vi "RobotSimulator.vi"() -> ()   [LabVIEW 2018]
uses:
  Robot-Project/Drive/Implementation/Drive Setpoints.ctl
  Robot-Project/Drive/Implementation/Drive Operations.ctl
  Controls/PurePursuit/RobotNeededPathData.ctl
  Robot-Project/Drive/DriveState.ctl
  <extravilib>/ChannelInstances/Lossy Stream-c(dbl,dbl,dbl,c(dbl,dbl))/Write With Abort.vi
  <extravilib>/ChannelInstances/Lossy Stream-c(dbl,dbl,dbl,c(dbl,dbl))/Read With Abort.vi
  <extravilib>/ChannelInstances/Lossy Stream-c(dbl,dbl,dbl,c(dbl,dbl))/Endpoint.vi
  <extravilib>/ChannelInstances/Lossy Stream-c(dbl,dbl,dbl,c(dbl,dbl))/EndpointRead.vi
  Robot-Project/Drive/Implementation/Drive Published Globals.vi
  <extravilib>/ChannelInstances/Lossy Stream-c(dbl,dbl,dbl,c(dbl,dbl))/Instantiate.vi
  <extravilib>/ChannelInstances/Lossy Stream-c(dbl,dbl,dbl,c(dbl,dbl))/)Channel.vi
  <resource>/ChannelSupport/_ChannelSupport/WaitIfNeeded.vi
  <vilib>/addons/control/pid/pid.llb/PID (DBL).vi
  Robot-Project/Configuration/Constants.vi
  <vilib>/addons/control/pid/NI_PID_pid.lvlib
  <extravilib>/ChannelInstances/Lossy Stream-c(dbl,dbl,dbl,c(dbl,dbl)).lvlib
panel:
  in  "Path":cluster{dbl, dbl}[](array[cluster])
  in  "Angle Addition":dbl(slide) scale=-180.0..180.0
  in  "Target":cluster{dbl, dbl}={200.0, 200.0}
  out "Current\nCmd":string="Started at  14:51:47.884\nDefault: Reserve,  L 0.0, R 0.0, D 0.000000"
  in  "Go":bool
  out "Loop Iterations":i32
  in  "Gains 2":T1={"Gains"={"FFV"=0.0055, "FFA"=0.0025, "Vel PID"={"P"=0.05, "I"=0.0, "D"=0.0}}, "Pos PID"={"P"=0.05, "I"=0.0, "D"=0.0}, "MinVoltage"=0.0, "Effective Trackwidth"=29.0, "Effective Trackwidth CCW"=29.0} {"Pos PID"."D" format="%.3f"; "Pos PID"."I" format="%.3f"; "Pos PID"."P" format="%.3f"; "Gains"."Vel PID"."D" format="%.3f"; "Gains"."Vel PID"."I" format="%.3f"; "Gains"."Vel PID"."P" format="%.3f"}
  out "Graph":cluster{cluster{"x":dbl, "y":dbl}[]}[](graph)=[{[]}, {[{"x"=19.5, "y"=127.60329985652797}, {"x"=31.499289530461766, "y"=127.73387843115106}]}, {[{"x"=0.0, "y"=0.0}]}, {[{"x"=19.5, "y"=127.60329985652797}, {"x"=19.5, "y"=127.60329985652797}, {"x"=19.5, "y"=127.60329985652797}, {"x"=19.5, "y"=127.60329985652797}, {"x"=19.5, "y"=127.60329985652797}, {"x"=19.5, "y"=127.60329985652797}, {"x"=19.5, "y"=127.60329985652797}, {"x"=19.5, "y"=127.60329985652797}, {"x"=19.5, "y"=127.60329985652797}, {"x"=19.5, "y"=127.60329985652797}, {"x"=19.5, "y"=127.60329985652797}, {"x"=19.5, "y"=127.60329985652797}, {"x"=19.5, "y"=127.60329985652797}, {"x"=19.5, "y"=127.60329985652797}, {"x"=19.5, "y"=127.60329985652797}, {"x"=19.5, "y"=127.60329985652797}, {"x"=19.5, "y"=127.60329985652797}, {"x"=19.5, "y"=127.60329985652797}, {"x"=19.5, "y"=127.60329985652797}, {"x"=19.5, "y"=127.60329985652797}, {"x"=19.5, "y"=127.60329985652797}, {"x"=19.5, "y"=127.60329985652797}, {"x"=19.5, "y"=127.60329985652797}, {"x"=19.5, "y"=127.60329985652797}, {"x"=19.5, "y"=127.60329985652797}, {"x"=19.5, "y"=127.60329985652797}, {"x"=19.5, "y"=127.60329985652797}, {"x"=19.5, "y"=127.60329985652797}, {"x"=19.5, "y"=127.60329985652797}, {"x"=19.5, "y"=127.60329985652797}, {"x"=19.5, "y"=127.60329985652797}]}, {[{"x"=inf, "y"=nan}, {"x"=inf, "y"=nan}, {"x"=inf, "y"=nan}, {"x"=inf, "y"=nan}, {"x"=inf, "y"=nan}, {"x"=inf, "y"=nan}, {"x"=inf, "y"=nan}, {"x"=inf, "y"=nan}, {"x"=nan, "y"=nan}, {"x"=nan, "y"=nan}, {"x"=nan, "y"=nan}, {"x"=nan, "y"=nan}, {"x"=nan, "y"=nan}, {"x"=nan, "y"=nan}, {"x"=nan, "y"=nan}, {"x"=nan, "y"=nan}, {"x"=nan, "y"=-inf}, {"x"=nan, "y"=-inf}, {"x"=nan, "y"=-inf}, {"x"=nan, "y"=-inf}, {"x"=nan, "y"=-inf}, {"x"=nan, "y"=-inf}, {"x"=nan, "y"=-inf}, {"x"=inf, "y"=-inf}, {"x"=inf, "y"=-inf}, {"x"=inf, "y"=-inf}, {"x"=inf, "y"=-inf}, {"x"=inf, "y"=-inf}, {"x"=inf, "y"=-inf}, {"x"=inf, "y"=-inf}, {"x"=inf, "y"=-inf}]}]
  out "Right Output":dbl
  out "Left Output":dbl
  in  "Config":T2={"Gear Reduction"=8.7, "Wheel Radius (m)"=0.076, "# Motors"=3, "coeff of friction"=0.1, "Mass (kg)"=55.0, "Motor"={"Ke (V)"=0.0183, "R (ohms)"=0.14, "KT (Nm/A)"=0.0183, "Tf (Nm)"=0.015}}
  in  "Position":dbl=3.0
  in  "Gains":T3={"FFV"=0.0059, "FFA"=0.0019, "Vel PID"={"P"=0.01, "I"=0.0, "D"=0.0}}
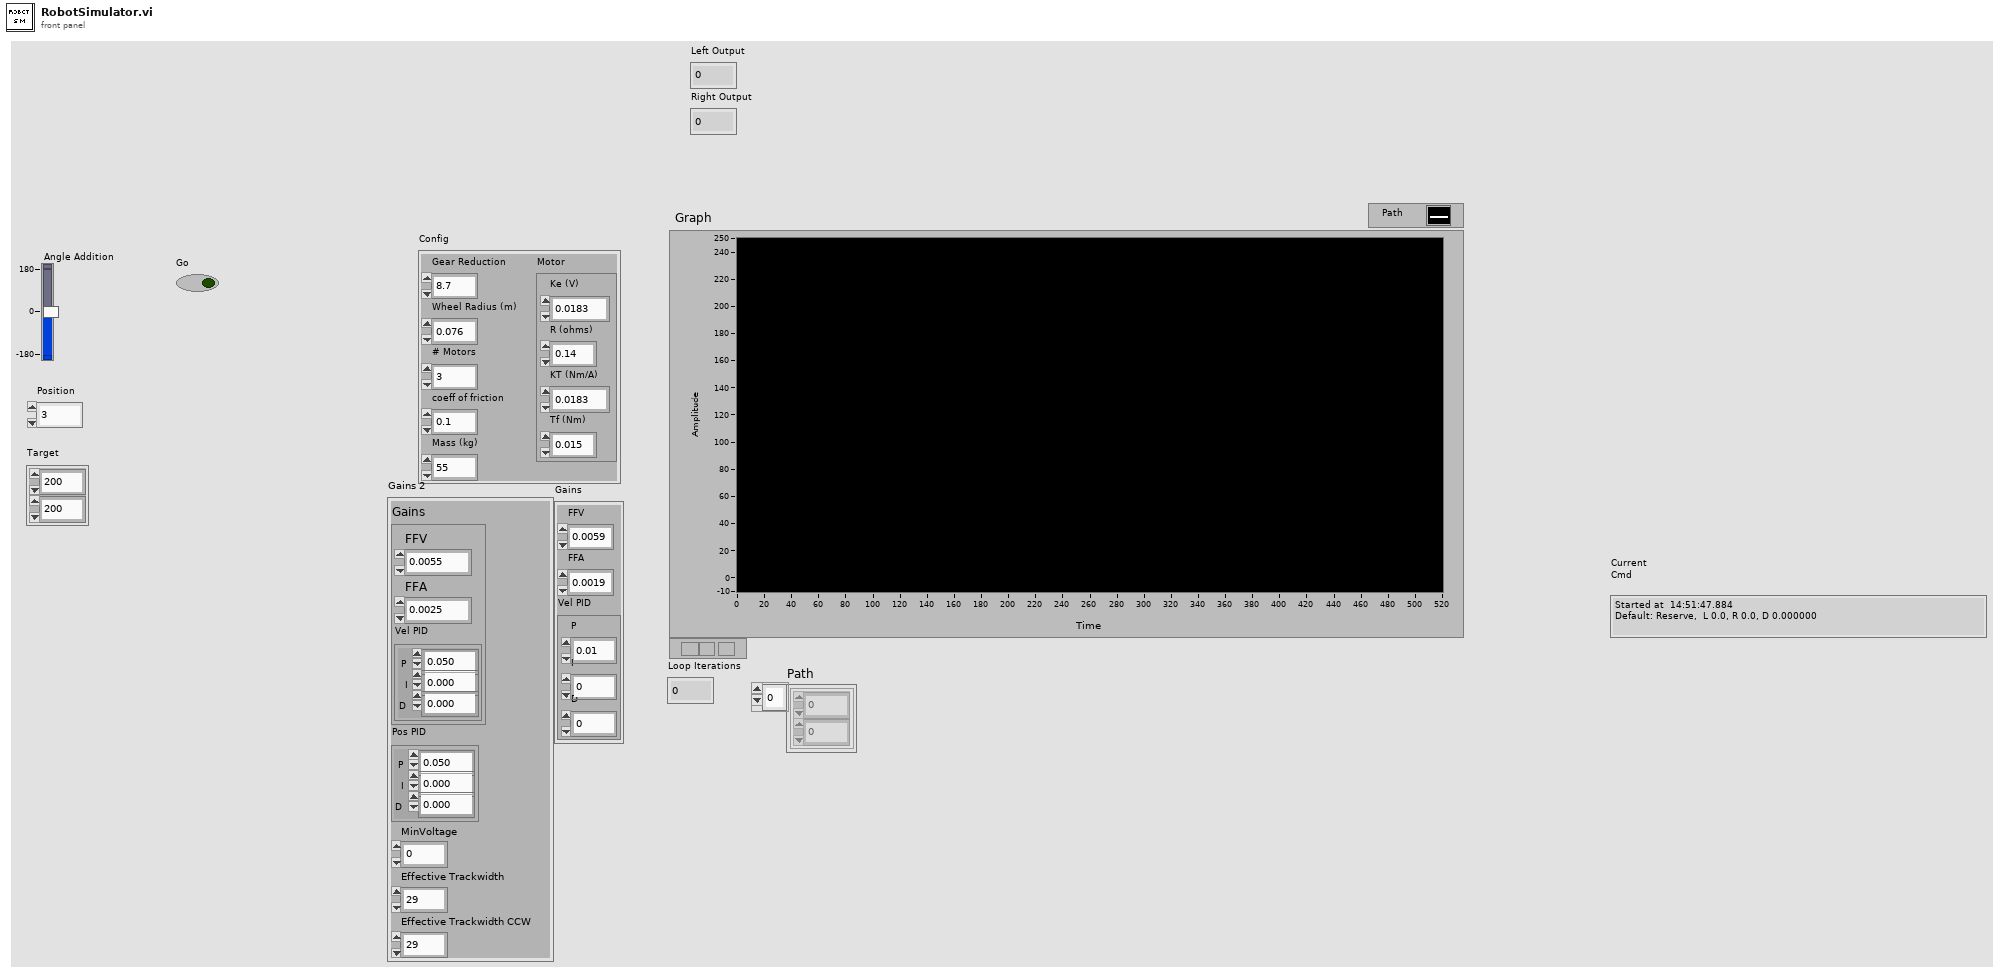
[diagram p1: front panel]
types:
  T1 = cluster{"Gains":cluster{"FFV":dbl, "FFA":dbl, "Vel PID":cluster{"P":dbl, "I":dbl, "D":dbl}}, "Pos PID":cluster{"P":dbl, "I":dbl, "D":dbl}, "MinVoltage":dbl, "Effective Trackwidth":dbl, "Effective Trackwidth CCW":dbl}
  T2 = cluster{"Gear Reduction":dbl, "Wheel Radius (m)":dbl, "# Motors":u32, "coeff of friction":dbl, "Mass (kg)":dbl, "Motor":cluster{"Ke (V)":dbl, "R (ohms)":dbl, "KT (Nm/A)":dbl, "Tf (Nm)":dbl}}
  T3 = cluster{"FFV":dbl, "FFA":dbl, "Vel PID":cluster{"P":dbl, "I":dbl, "D":dbl}}
  T4 = typedef "Drive Setpoints.ctl" = cluster{"Operation":T5, "Left Speed":dbl, "Right Speed":dbl, "Duration":dbl, "Speed":dbl, "Start Angle":dbl, "Target Angle":dbl, "Distance (inch)":dbl, "Start Point (inch)":dbl, "RobotNeededPathData":T6, "Start Point 2":dbl}
  T5 = typedef "Drive Operations.ctl" = enum16{"Reserve", "Read Current", "Immediate", "Drive for Time", "Drive for Distance", "Turn to Angle", "Drive Path"}
  T6 = typedef "RobotNeededPathData.ctl" = cluster{"Path":cluster{dbl, dbl}[], "MaxVel":dbl, "MaxAccel":dbl, "Backwards?":bool, "PointSpacing":dbl, "LookaheadDist":dbl, "Speed/Curve":dbl, "SlowDistanceAtEnd":dbl, "SlowSpeed":dbl, "MaxDeAccel":dbl}
  T7 = typedef "Command Status Info.ctl" = cluster{"Name":string, "Status":T8, "notifier out":T9}
  T8 = typedef "Completion Status.ctl" = enum16{"Successful", "Aborted", "Incomplete"}
  T9 = typedef "Completion Notifier.ctl" = refnum<notifier>
  T10 = cluster{"SubSystem Data":T4, cluster{"Start Time (ms)":u32, "Iterations":i32}, cluster{"Command Info":T7, "Description":string, "Default Command":T4, "queue out":refnum<queue>, "Subsystem Name":string}}
  T11 = typedef "DriveState.ctl" = enum16{"None", "Initial Turn", "Follow Path"}
  T12 = cluster{"LeftVel":dbl, "RightVel":dbl, "Yaw":dbl, "Pos":cluster{"X":dbl, "Y":dbl}}
  T13 = typedef "Lossy Stream-c(dbl,dbl,dbl,c(dbl,dbl)).lvlib/)Channel.ctl" = refnum<queue>
  T14 = cluster{"proportional gain (Kc)":dbl, "integral time (Ti, min)":dbl, "derivative time (Td, min)":dbl}
  T15 = cluster{"Angle":dbl, "Angular vel":dbl, "Left Distance":dbl, "Left vel":dbl, "Right Distance":dbl, "Right vel":dbl}
  T16 = cluster{"LeftDistance":dbl, "RightDistance":dbl, "LeftVelocity":dbl, "RightVelocity":dbl, "Angle":dbl, "Location":cluster{dbl, dbl}}
  T17 = cluster{"dx/dt":dbl, "dx/dt":dbl, "Yaw":dbl, cluster{dbl, dbl}}
  T18 = cluster{"SubSystem Data":T4, cluster{"Start Time (ms)":u32, "Iterations":i32}, "Default Command Arguments":cluster{"Command Info":T7, "Description":string, "Default Command":T4, "queue out":refnum<queue>, "Subsystem Name":string}}
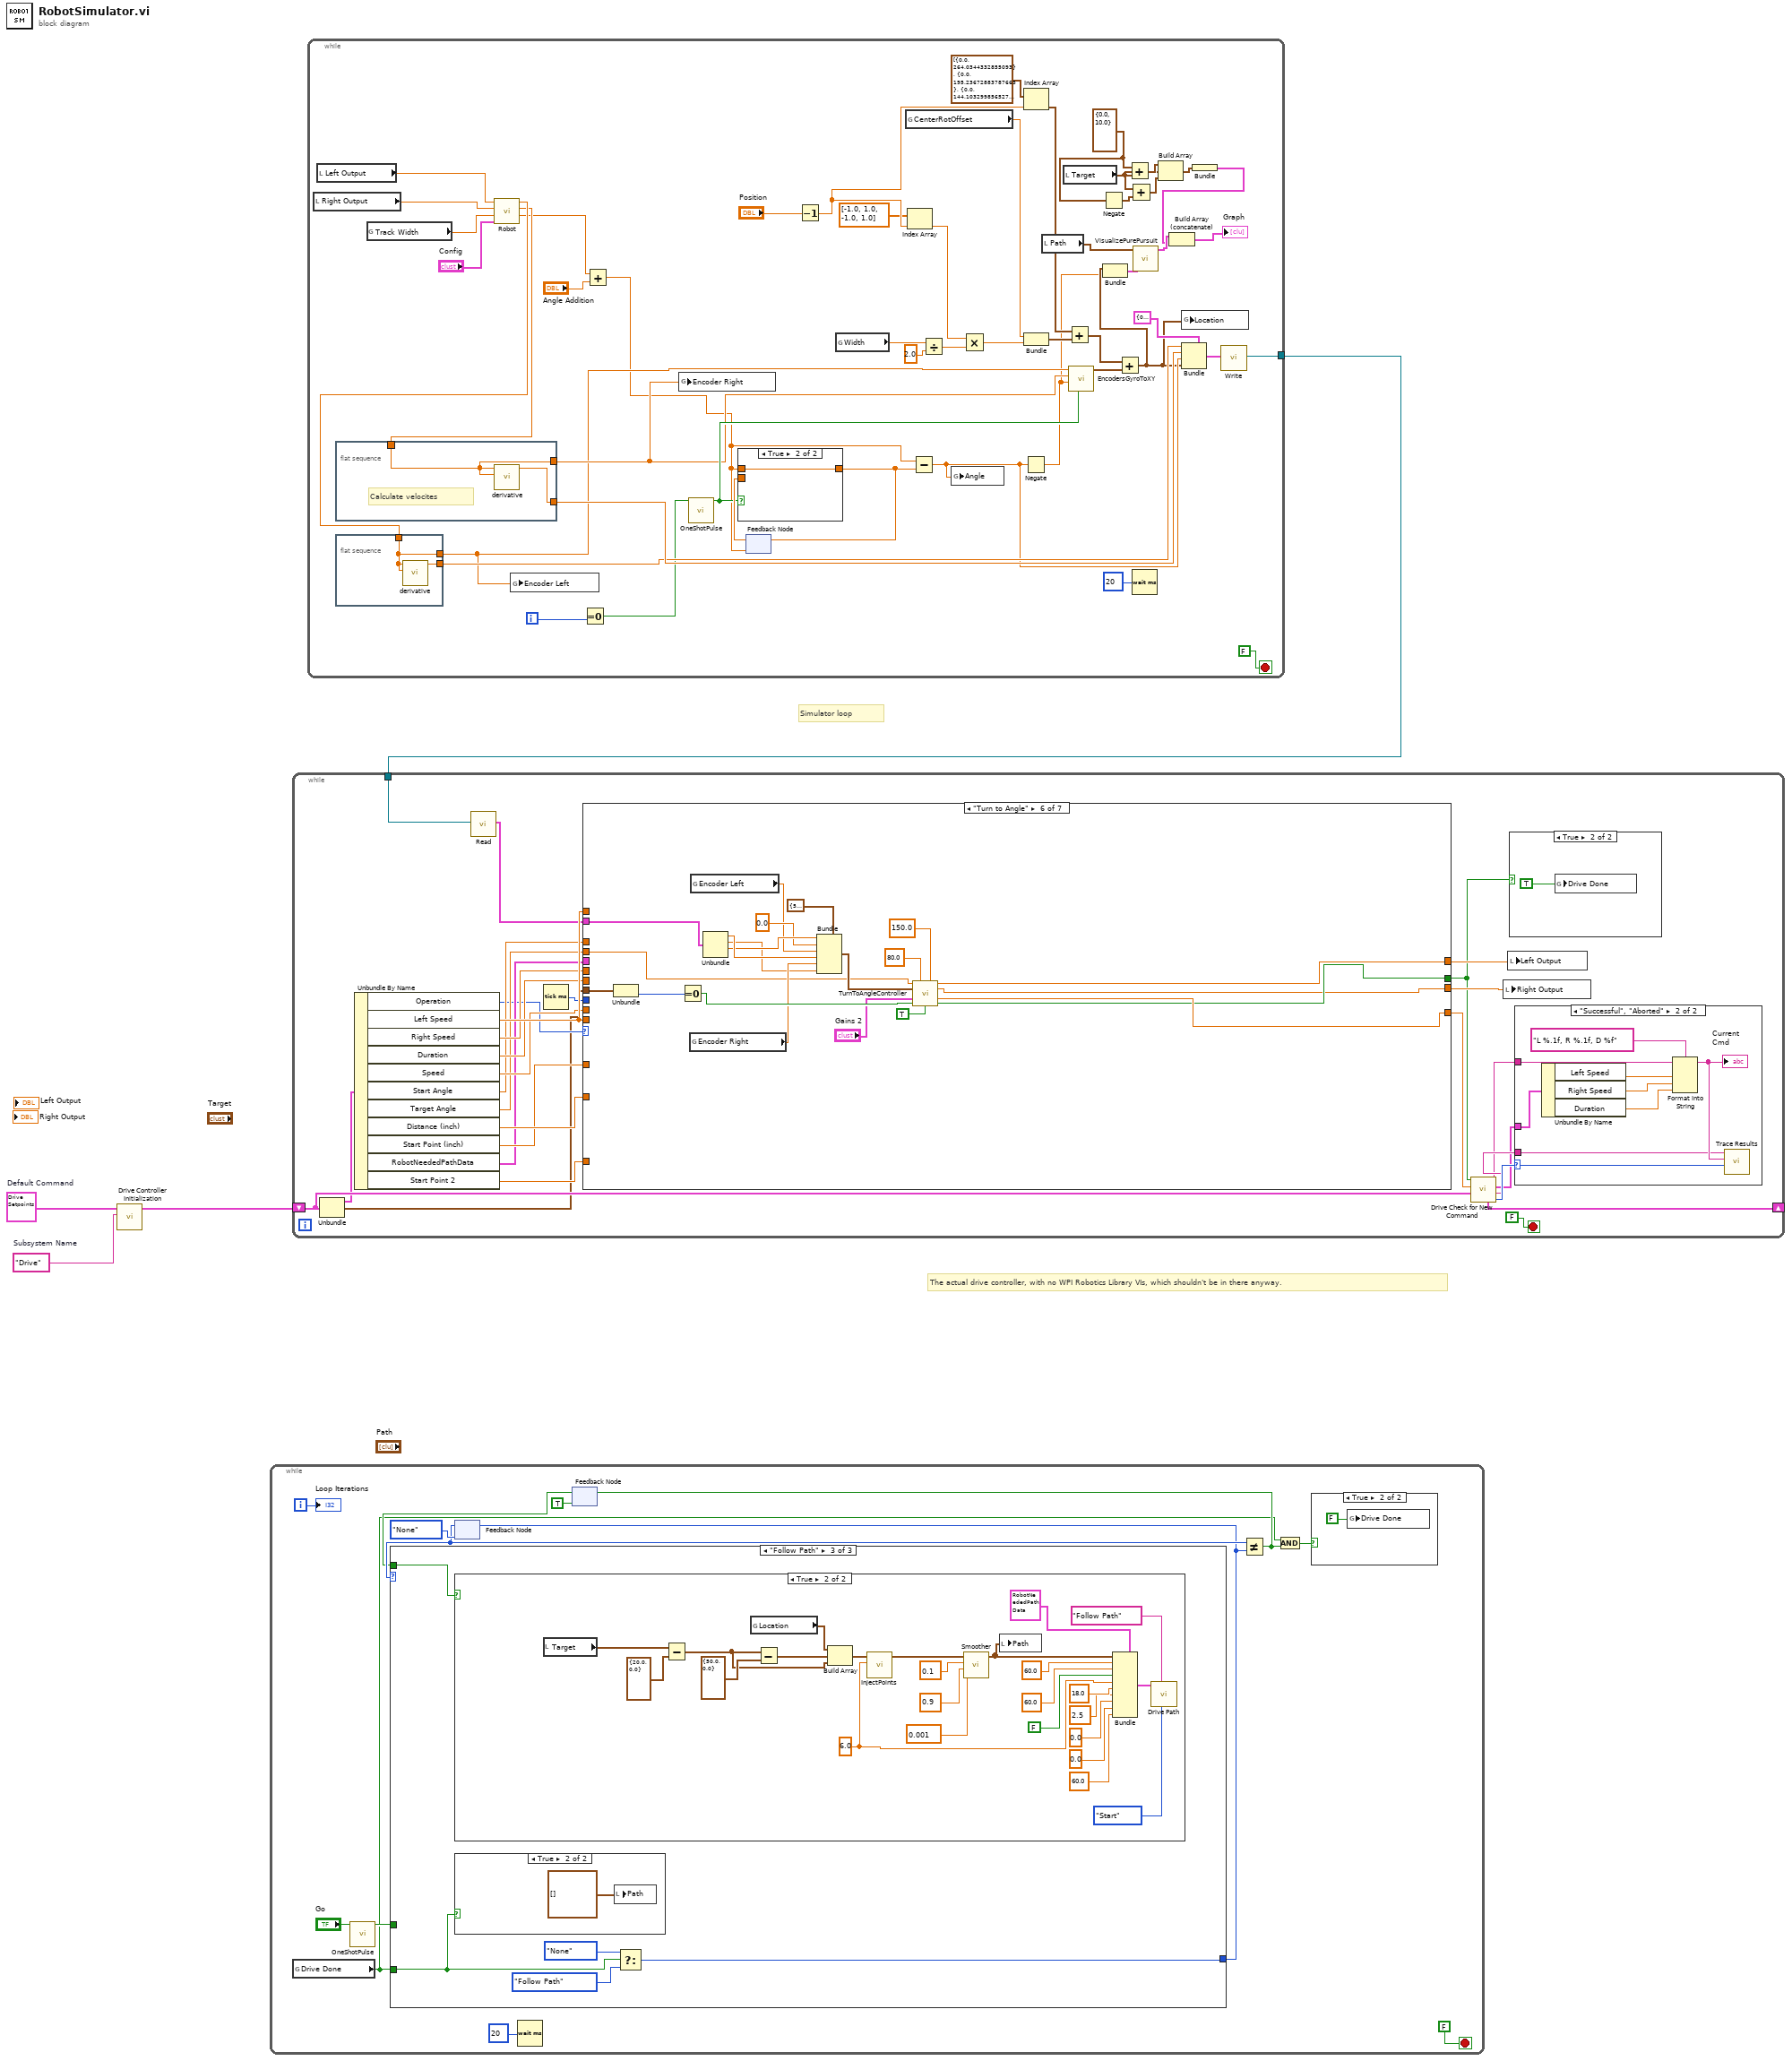
[diagram p0: block diagram]
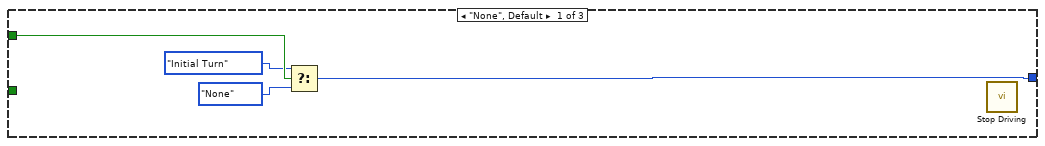
[diagram p3: hidden frame]
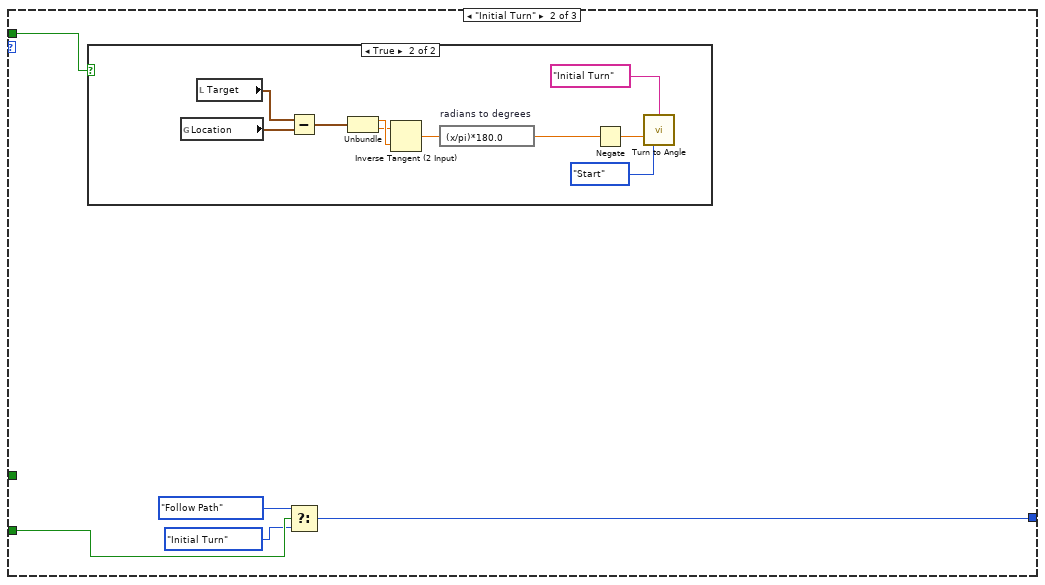
[diagram p4: hidden frame]
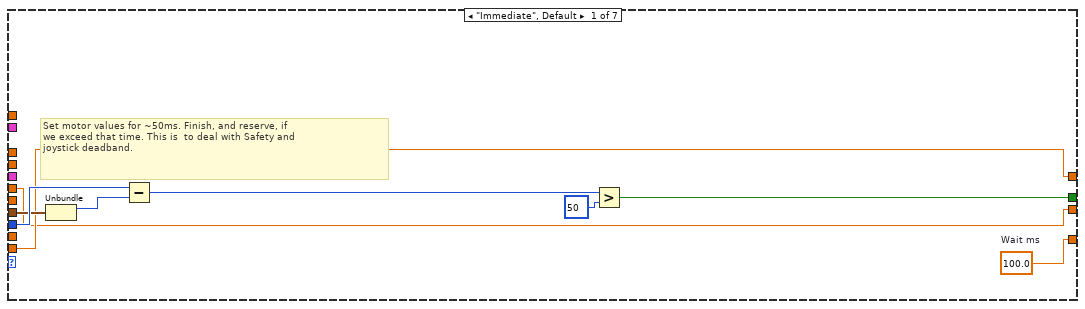
[diagram p11: hidden frame]
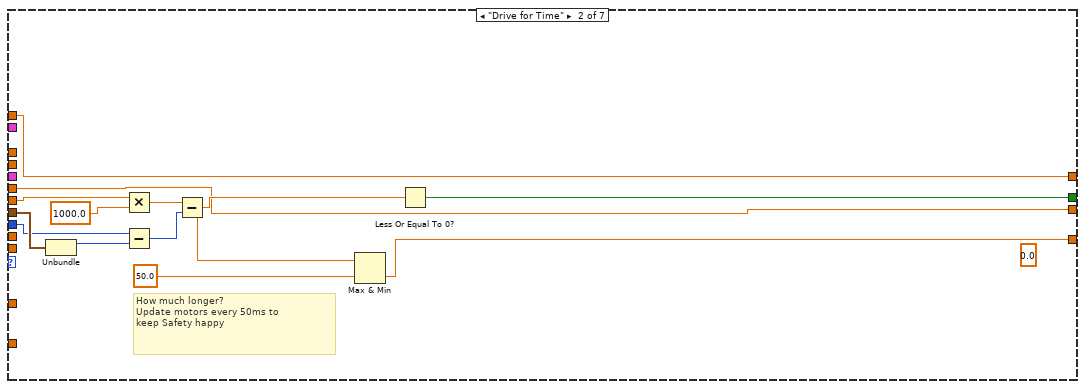
[diagram p12: hidden frame]
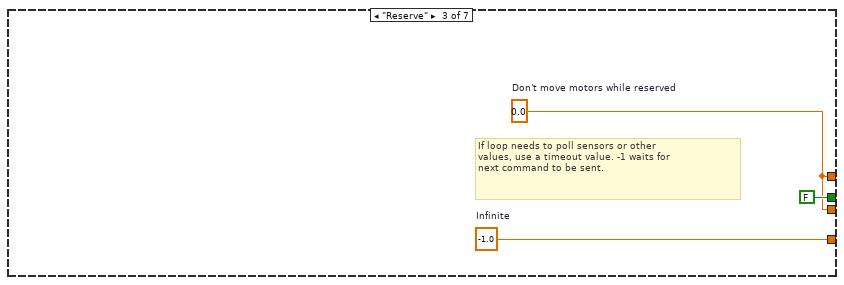
[diagram p13: hidden frame]
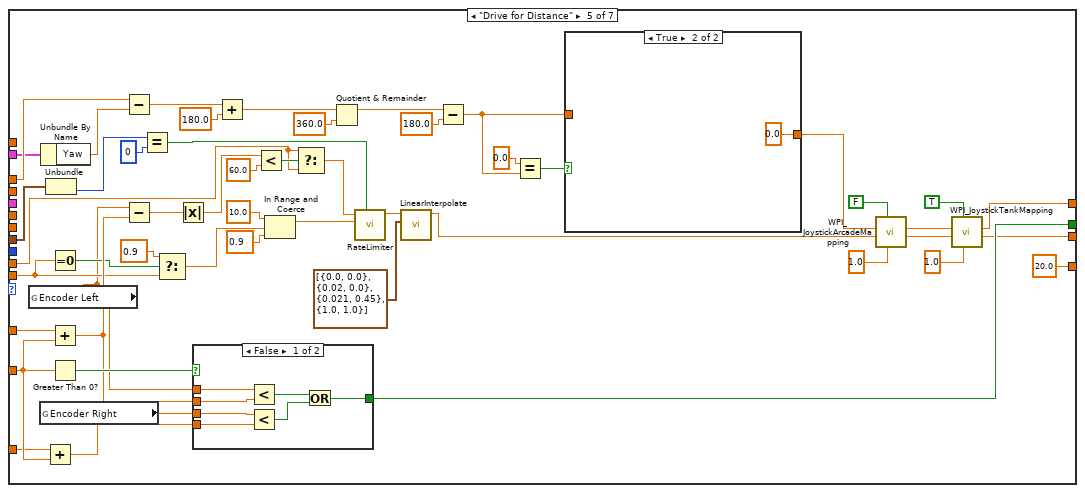
[diagram p15: hidden frame]
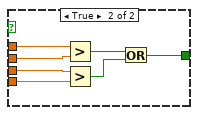
[diagram p16: hidden frame]
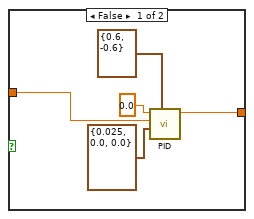
[diagram p17: hidden frame]
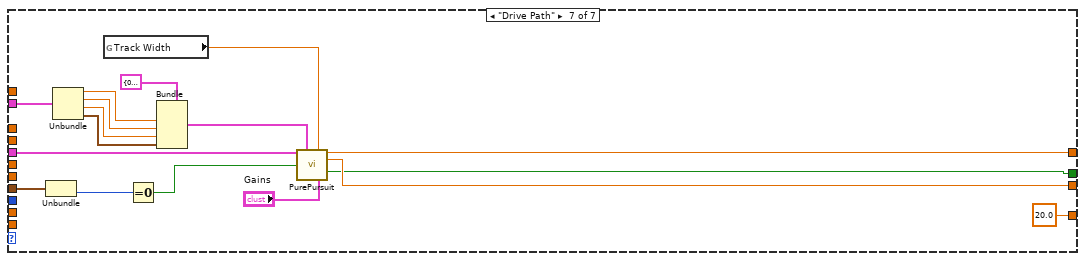
[diagram p18: hidden frame]
diagram:
  w3 = T4 {"Operation"=enum."Reserve", "Left Speed"=0.0, "Right Speed"=0.0, "Duration"=0.0, "Speed"=0.0, "Start Angle"=0.0, "Target Angle"=0.0, "Distance (inch)"=0.0, "Start Point (inch)"=0.0, "RobotNeededPathData"={"Path"=[], "MaxVel"=0.0, "MaxAccel"=0.0, "Backwards?"=FALSE, "PointSpacing"=0.0, "LookaheadDist"=0.0, "Speed/Curve"=1.8, "SlowDistanceAtEnd"=12.0, "SlowSpeed"=15.0, "MaxDeAccel"=0.0}, "Start Point 2"=0.0}  # Default Command
  w4 = "Drive"  # Subsystem Name
  # "Simulator loop"
  # "The actual drive controller, with no WPI Robotics Library VIs, which shouldn't be in there anyway."
  n1 = call "Drive Controller Initialization.vi"("Subsystem Name"=w4, "Default Command"=w3) -> ("Current Command"=w2:T10)  [unwired: 9 in]
  n2 = while {
    i -> [w15]
    stop <- FALSE stop-if-true
    n3 = global read "Drive Published Globals.vi" "Drive Done"() -> (w5:bool)
    n4 = call "OneShotPulse.vi"("Input"="Go") -> ("Output"=w12:bool)  [unwired: 10 in]
    n5 = feedback #1(DriveState."None" ("State")) -> (w11:T11)
    n6 = Wait (ms)(milliseconds to wait=u32 20) -> ()  [unwired: 1 out]
    n7 = feedback #2(TRUE) -> (w8:bool)
    n8 = case shown="\"Follow Path\"" w11 {
      tunnel: w12 -> [w22 _ _]
      tunnel: [w20 w25 w41] -> w10
      tunnel: w8 -> [_ w27 w42]
      tunnel: w5 -> [_ w26 w38]
      frame "None", Default {
        n9 = Select(t=DriveState."Initial Turn", s=w22, f=DriveState."None" ("State")) -> (s? t:f=w20:T11)
        n10 = call "Stop Driving.vi"() -> ()  [unwired: 11 in, 1 out]
      }
      frame "Initial Turn" {
        n11 = case shown="True" w27 {
          frame False {
          }
          frame True {
            n12 = global read "Drive Published Globals.vi" "Location"() -> (w35:cluster{dbl, dbl})
            n13 = local read "Target"() -> (w34:cluster{dbl, dbl})
            n14 = Subtract(x=w34, y=w35) -> (x-y=w33:cluster{dbl, dbl})
            n15 = Unbundle(w33) -> (w32:dbl, w31:dbl)
            n16 = Inverse Tangent (2 Input)(1:w32, 2:w31) -> (0:w30:dbl)
            n17 = expression code="(x/pi)*180.0" "radians to degrees"(w30) -> (w29:dbl)
            n18 = Negate(x=w29) -> (-x=w28:dbl)
            n19 = call "Turn to Angle.vi"("Description"="Initial Turn", "Target Angle"=w28, "Synchronication"=enum16{"Start", "Wait"}."Start") -> ()  [unwired: 12 in, 1 out]
          }
        }
        n20 = Select(t=DriveState."Follow Path" ("State"), s=w26, f=DriveState."Initial Turn" ("State")) -> (s? t:f=w25:T11)
      }
      frame "Follow Path" {
        n21 = case shown="True" w42 {
          frame False {
          }
          frame True {
            w53 = 6.0 ("Distance")
            n22 = local read "Target"() -> (w67:cluster{dbl, dbl})
            n23 = Subtract(x=w67, y=cluster{dbl, dbl} {20.0, 0.0}) -> (x-y=w62:cluster{dbl, dbl})
            n24 = global read "Drive Published Globals.vi" "Location"() -> (w64:cluster{dbl, dbl})
            n25 = Subtract(x=w62, y=cluster{dbl, dbl} {50.0, 0.0}) -> (x-y=w63:cluster{dbl, dbl})
            n26 = Build Array(w64, w63, w62) -> (w58:cluster{dbl, dbl}[])
            n27 = call "InjectPoints.vi"("Spacing"=w53, "Path"=w58) -> ("Path out"=w45:cluster{dbl, dbl}[])  [unwired: 9 in]
            n28 = call "Smoother.vi"("tolerance"=0.001, "B"=0.9, "A"=0.1, "Path"=w45) -> ("SmoothPath"=w44:cluster{dbl, dbl}[])  [unwired: 7 in]
            n29 = local write "Path"(w44) -> ()
            n30 = Bundle(cluster=T6 {"Path"=[], "MaxVel"=0.0, "MaxAccel"=0.0, "Backwards?"=FALSE, "PointSpacing"=0.0, "LookaheadDist"=0.0, "Speed/Curve"=1.8, "SlowDistanceAtEnd"=12.0, "SlowSpeed"=15.0, "MaxDeAccel"=0.0} ("Path"), "Path"=w44, "MaxVel"=60.0, "MaxAccel"=60.0, "Backwards?"=FALSE, "PointSpacing"=w53, "LookaheadDist"=18.0, "Speed/Curve"=2.5, "SlowDistanceAtEnd"=0.0, "SlowSpeed"=0.0, "MaxDeAccel"=60.0) -> (w47:T6)
            n31 = call "Drive Path.vi"("Synchronication"=enum16{"Start", "Wait"}."Start", "Description"="Follow Path", "Path"=w47) -> ()  [unwired: 8 in, 1 out]
          }
        }
        n32 = case shown="True" w38 {
          frame False {
          }
          frame True {
            n33 = local write "Path"(cluster{dbl, dbl}[] [] ("Path")) -> ()
          }
        }
        n34 = Select(t=DriveState."None" ("State"), s=w38, f=DriveState."Follow Path") -> (s? t:f=w41:T11)
      }
    }
    n35 = feedback-in #1(w10) -> ()
    n36 = Not Equal?(x=w11, y=w10) -> (x != y?=w7:bool)
    n37 = feedback-in #2(w7) -> ()
    n38 = And(x=w5, y=w7) -> (x .and. y?=w6:bool)
    n39 = case shown="True" w6 {
      frame False {
      }
      frame True {
        n40 = global write "Drive Published Globals.vi" "Drive Done"(FALSE ("Command Done")) -> ()
      }
    }
    "Loop Iterations" <- w15
  }
  n41 = while {
    tunnel: [w94] -> w1
    i -> [w93]
    stop <- FALSE stop-if-true
    w74 = cluster{dbl, dbl} {0.0, 10.0} ("x")
    n42 = local read "Right Output"() -> (w88:dbl)
    n43 = local read "Left Output"() -> (w87:dbl)
    n44 = flat-sequence {
      tunnel: [w125] -> w117
      tunnel: [w124] -> w100
      tunnel: w82 -> [w124]
      frame #0 {
        # "Calculate velocites"
        n45 = call "derivative.vi"("Starting value"=w124, "x"=w124) -> ("dx/dt"=w125:dbl)  [unwired: 9 in]
      }
    }
    n46 = flat-sequence {
      tunnel: [w121] -> w101
      tunnel: [w120] -> w99
      tunnel: w83 -> [w120]
      frame #0 {
        n47 = call "derivative.vi"("Starting value"=w120, "x"=w120) -> ("dx/dt"=w121:dbl)  [unwired: 9 in]
      }
    }
    n48 = global read "Constants.vi" "Track Width"() -> (w89:dbl)
    n49 = call "Robot.vi"("Config"="Config", "WheelBase"=w89, "Right Value"=w88, "Left Value"=w87) -> ("Angle"=w77:dbl, "Right Distance"=w82:dbl, "Left Distance"=w83:dbl)  [unwired: 5 in]
    n50 = global write "Drive Published Globals.vi" "Encoder Left"(w99) -> ()
    n51 = Equal To 0?(x=w93) -> (x = 0?=w92:bool)
    n52 = Add(x=w77, y="Angle Addition") -> (x+y=w75:dbl)
    n53 = global write "Drive Published Globals.vi" "Encoder Right"(w100) -> ()
    n54 = call "OneShotPulse.vi"("Input"=w92) -> ("Output"=w113:bool)  [unwired: 10 in]
    n55 = feedback #3(w75) -> (w114:dbl)
    n56 = case shown="True" w113 {
      tunnel: w75 -> [_ w123]
      tunnel: [w122 w123] -> w115
      tunnel: w114 -> [w122 _]
      frame False {
      }
      frame True {
      }
    }
    n57 = feedback-in #3(w115) -> ()
    n58 = Decrement(x="Position") -> (x-1=w109:dbl)
    n59 = global read "Constants.vi" "Width"() -> (w104:dbl)
    n60 = global read "Constants.vi" "CenterRotOffset"() -> (w102:dbl)
    n61 = Index Array(array=dbl[] [-1.0, 1.0, -1.0, 1.0], index=w109) -> (element=w110:dbl)
    n62 = Subtract(x=w75, y=w115) -> (x-y=w97:dbl)
    n63 = Divide(x=w104, y=2.0) -> (x/y=w105:dbl)
    n64 = global write "Drive Published Globals.vi" "Angle"(w97) -> ()
    n65 = Multiply(x=w110, y=w105) -> (x*y=w111:dbl)
    n66 = Negate(x=w97) -> (-x=w84:dbl)
    n67 = Index Array(array=cluster{dbl, dbl}[] [{0.0, 264.0344332855093}, {0.0, 195.23672883787663}, {0.0, 144.10329985652797}, {0.0, -0.0}] ("x*y"), index=w109) -> (element=w108:cluster{dbl, dbl})
    n68 = Bundle("CenterRotOffset"=w102, w111) -> (w112:cluster{"CenterRotOffset":dbl, dbl})  [unwired: 1 in]
    n69 = local read "Path"() -> (w69:cluster{dbl, dbl}[])
    n70 = local read "Target"() -> (w71:cluster{dbl, dbl})
    n71 = Add(x=w108, y=w112) -> (x+y=w98:cluster{dbl, dbl})
    n72 = call "EncodersGyroToXY.vi"("Reset"=w113, "Angle (degrees)"=w84, "Right Distance"=w100, "Left Distance"=w99) -> ("Location"=w116:cluster{dbl, dbl})  [unwired: 7 in]
    n73 = Negate(x=w74) -> (-x=w73:cluster{dbl, dbl})
    n74 = Add(x=w98, y=w116) -> (x+y=w86:cluster{dbl, dbl})
    n75 = Bundle(w86, w84) -> (w85:cluster{cluster{dbl, dbl}, dbl})  [unwired: 1 in]
    n76 = Add(x=w74, y=w71) -> (x+y=w72:cluster{dbl, dbl})
    n77 = Add(x=w71, y=w73) -> (x+y=w70:cluster{dbl, dbl})
    n78 = Wait (ms)(milliseconds to wait=u32 20) -> ()  [unwired: 1 out]
    n79 = call "VisualizePurePursuit.vi"("Robot"=w85, "Path"=w69) -> ("Graph"=w80:cluster{cluster{"x":dbl, "y":dbl}[]}[])  [unwired: 9 in]
    n80 = Build Array(w72, w71, w70) -> (w81:cluster{dbl, dbl}[])
    n81 = global write "Drive Published Globals.vi" "Location"(w86) -> ()
    n82 = Bundle(cluster=T12 {"LeftVel"=0.0, "RightVel"=0.0, "Yaw"=0.0, "Pos"={"X"=0.0, "Y"=0.0}} ("Robot"), "LeftVel"=w101, "RightVel"=w117, "Yaw"=w97, "Pos"=w86) -> (w95:T12)
    n83 = Bundle(w81) -> (w78:cluster{cluster{dbl, dbl}[]})  [unwired: 1 in]
    n84 = Build Array (concatenate)(w80, w78) -> (→"Graph":cluster{cluster{"x":dbl, "y":dbl}[]}[])
    n85 = call <extravilib>:"Write.vi"("element"=w95) -> ("channel"=w94:T13)  [unwired: 8 in, 2 out]
  }
  n86 = while {
    shift-right: [w152] -> _
    shift-left: w2 -> [w150]
    tunnel: w1 -> [w134]
    stop <- FALSE stop-if-true
    n87 = Unbundle(w150) -> ("SubSystem Data"=w136:T4, w135:cluster{"Start Time (ms)":u32, "Iterations":i32})  [unwired: 1 out]
    n88 = Unbundle By Name(w136) -> ("Operation"=w139:T5, "Left Speed"=w149:dbl, "Right Speed"=w148:dbl, "Duration"=w147:dbl, "Speed"=w146:dbl, "Start Angle"=w145:dbl, "Target Angle"=w144:dbl, "Distance (inch)"=w143:dbl, "Start Point (inch)"=w142:dbl, "RobotNeededPathData"=w141:T6, "Start Point 2"=w140:dbl)
    n89 = call <extravilib>:"Read.vi"("channel"=w134) -> ("element"=w133:T17)  [unwired: 5 in, 5 out]
    n90 = Tick Count (ms)() -> (millisecond timer value=w138:u32)
    n91 = case shown="\"Turn to Angle\"" w139 {
      tunnel: [w171 w175 w187 _ 20.0 ("Infinite") w276 20.0 ("Infinite")] -> w137
      tunnel: [w166 w179 FALSE ("ignore previous (F)") _ w229 w275 w293] -> w126
      tunnel: w135 -> [w165 w181 _ _ w212 w279 w283]
      tunnel: w138 -> [w167 w178 _ _ _ _ _]
      tunnel: [w164 w173 w185 _ w217 w274 w295] -> w127
      tunnel: [w163 w172 w185 _ w218 w273 w294] -> w132
      tunnel: w146 -> [_ _ _ _ w202 _ _]
      tunnel: w143 -> [_ _ _ _ w201 _ _]
      tunnel: w147 -> [_ w174 _ _ _ _ _]
      tunnel: w149 -> [w164 _ _ _ w196 _ _]
      tunnel: w148 -> [w163 w172 _ _ _ _ _]
      tunnel: w145 -> [_ _ _ _ w224 _ _]
      tunnel: w144 -> [_ _ _ _ _ w262 _]
      tunnel: w142 -> [_ _ _ _ w223 _ _]
      tunnel: w149 -> [_ w173 _ _ _ _ _]
      tunnel: w141 -> [_ _ _ _ _ _ w296]
      tunnel: w133 -> [_ _ _ _ w191 w270 w287]
      tunnel: w140 -> [_ _ _ _ w200 _ _]
      frame "Immediate", Default {
        w171 = 100.0  # Wait ms
        # "Set motor values for ~50ms. Finish, and reserve, if\nwe exceed that time. This is  to deal with Safety and\njoystick deadband."
        n92 = Unbundle(w165) -> ("Start Time (ms)"=w168:u32)  [unwired: 1 out]
        n93 = Subtract(x=w167, y=w168) -> (x-y=w169:u32)
        n94 = Greater?(x=w169, y=u8 50 ("Left Motor")) -> (0:w166:bool)
      }
      frame "Drive for Time" {
        (unwired) 0.0 ("output")
        # "How much longer?\nUpdate motors every 50ms to\nkeep Safety happy"
        n95 = Unbundle(w181) -> ("Start Time (ms)"=w180:u32)  [unwired: 1 out]
        n96 = Multiply(x=w174, y=1000.0) -> (x*y=w183:dbl)
        n97 = Subtract(x=w178, y=w180) -> (x-y=w184:u32)
        n98 = Subtract(x=w183, y=w184) -> (x-y=w177:dbl)
        n99 = Max & Min(x=w177, y=50.0) -> (min(x,y)=w175:dbl)  [unwired: 1 out]
        n100 = Less Or Equal To 0?(x=w177) -> (x <= 0?=w179:bool)
      }
      frame "Reserve" {
        w185 = 0.0  # Don't move motors while reserved
        w187 = -1.0  # Infinite
        # "If loop needs to poll sensors or other\nvalues, use a timeout value. -1 waits for\nnext command to be sent."
      }
      frame "Read Current" {
      }
      frame "Drive for Distance" {
        n101 = global read "Drive Published Globals.vi" "Encoder Left"() -> (w189:dbl)
        n102 = global read "Drive Published Globals.vi" "Encoder Right"() -> (w188:dbl)
        n103 = Unbundle By Name(w191) -> ("Yaw"=w190:dbl)
        n104 = Add(x=w200, y=w201) -> (x+y=w199:dbl)
        n105 = Unbundle(w212) -> ("Iterations"=w211:i32)  [unwired: 1 out]
        n106 = Equal To 0?(x=w196) -> (x = 0?=w198:bool)
        n107 = Add(x=w223, y=w201) -> (x+y=w208:dbl)
        n108 = Greater Than 0?(x=w201) -> (x > 0?=w222:bool)
        n109 = Subtract(x=w224, y=w190) -> (x-y=w231:dbl)
        n110 = Subtract(x=w189, y=w208) -> (x-y=w207:dbl)
        n111 = Equal?(x=w211, y=0) -> (x = y?=w209:bool)
        n112 = Select(t=0.9, s=w198, f=w196) -> (s? t:f=w195:dbl)
        n113 = Absolute Value(x=w207) -> (abs(x)=w206:dbl)
        n114 = case shown="False" w222 {
          tunnel: w189 -> [w244 w252]
          tunnel: w208 -> [w245 w251]
          tunnel: [w242 w246] -> w229
          tunnel: w199 -> [w240 w250]
          tunnel: w188 -> [w241 w249]
          frame False {
            n115 = Less?(x=w244, y=w245) -> (x < y?=w243:bool)
            n116 = Less?(x=w241, y=w240) -> (x < y?=w239:bool)
            n117 = Or(x=w243, y=w239) -> (x .or. y?=w242:bool)
          }
          frame True {
            n118 = Greater?(x=w252, y=w251) -> (0:w248:bool)
            n119 = Greater?(x=w249, y=w250) -> (0:w247:bool)
            n120 = Or(x=w248, y=w247) -> (x .or. y?=w246:bool)
          }
        }
        n121 = Add(x=w231, y=180.0) -> (x+y=w235:dbl)
        n122 = Less?(x=w206, y=60.0) -> (x < y?=w204:bool)
        n123 = In Range and Coerce(upper limit=10.0, x=w195, lower limit=0.9) -> (coerced(x)=w192:dbl)  [unwired: 1 out]
        n124 = Select(t=w202, s=w204, f=w202) -> (s? t:f=w203:dbl)
        n125 = Quotient & Remainder(x=w235, y=360.0) -> (x-y*floor(x/y)=w233:dbl)  [unwired: 1 out]
        n126 = call "RateLimiter.vi"("Reset"=w209, "Max dx/dt"=w192, "Input"=w203) -> ("Output"=w220:dbl)  [unwired: 8 in]
        n127 = call "LinearInterpolate.vi"("Points"=cluster{"X":dbl, "Y":dbl}[] [{"X"=0.0, "Y"=0.0}, {"X"=0.02, "Y"=0.0}, {"X"=0.021, "Y"=0.45}, {"X"=1.0, "Y"=1.0}], "Value"=w220) -> ("Output"=w221:dbl)  [unwired: 9 in]
        n128 = Subtract(x=w233, y=180.0) -> (x-y=w230:dbl)
        n129 = Equal?(x=0.0, y=w230) -> (x = y?=w238:bool)
        n130 = case shown="True" w238 {
          tunnel: [w253 0.0] -> w225
          tunnel: w230 -> [w254 _]
          frame False {
            n131 = call-poly <vilib>:"PID.vi"("output range"=cluster{"output high":dbl, "output low":dbl} {"output high"=0.6, "output low"=-0.6}, "PID gains"=T14 {"proportional gain (Kc)"=0.025, "integral time (Ti, min)"=0.0, "derivative time (Td, min)"=0.0}, "process variable"=w254, "setpoint"=0.0) -> ("output"=w253:dbl)  [unwired: 6 in, 1 out]
          }
          frame True {
          }
        }
        n132 = call <vilib>:"WPI_JoystickArcadeMapping.vi"("Max Output"=1.0, "Square Inputs"=FALSE, "Y axis value"=w221, "X axis value"=w225) -> ("Right Motor Value"=w216:dbl, "Left Motor Value"=w215:dbl)  [unwired: 6 in]
        n133 = call <vilib>:"WPI_JoystickTankMapping.vi"("Max Output"=1.0, "Square Inputs"=TRUE, "Right axis value"=w216, "Left axis value"=w215) -> ("Right Motor Value"=w218:dbl, "Left Motor Value"=w217:dbl)  [unwired: 6 in]
      }
      frame "Turn to Angle" {
        n134 = Unbundle(w279) -> ("Iterations"=w278:i32)  [unwired: 1 out]
        n135 = Equal To 0?(x=w278) -> (x = 0?=w277:bool)
        n136 = global read "Drive Published Globals.vi" "Encoder Right"() -> (w265:dbl)
        n137 = global read "Drive Published Globals.vi" "Encoder Left"() -> (w266:dbl)
        n138 = Unbundle(w270) -> ("dx/dt"=w269:dbl, "dx/dt"=w260:dbl, "Yaw"=w268:dbl)  [unwired: 1 out]
        n139 = Bundle(cluster=T15 {"Angle"=548.1299999999924, "Angular vel"=0.49263510517714687, "Left Distance"=26.0882735, "Left vel"=0.0, "Right Distance"=-234.57467250000002, "Right vel"=0.0} ("Robot"), "Angle"=w268, "Angular vel"=0.0, "Left Distance"=w266, "Left vel"=w269, "Right Distance"=w265, "Right vel"=w260) -> (w272:T15)
        n140 = call "TurnToAngleController.vi"("TargetAngle"=w262, "MaxVel"=80.0, "MaxAccel"=150.0, "Robot"=w272, "Gains"="Gains 2", "Reset"=w277, "GoSmallestDistance"=TRUE) -> ("LeftPower"=w274:dbl, "RightPower"=w273:dbl, "Delay"=w276:dbl, "Done"=w275:bool)  [unwired: 2 in, 3 out]
      }
      frame "Drive Path" {
        n141 = Unbundle(w283) -> ("Iterations"=w284:i32)  [unwired: 1 out]
        n142 = Unbundle(w287) -> ("dx/dt"=w291:dbl, "dx/dt"=w290:dbl, "Yaw"=w289:dbl, w288:cluster{dbl, dbl})
        n143 = global read "Constants.vi" "Track Width"() -> (w282:dbl)
        n144 = Equal To 0?(x=w284) -> (x = 0?=w285:bool)
        n145 = Bundle(cluster=T16 {"LeftDistance"=0.0, "RightDistance"=0.0, "LeftVelocity"=0.0, "RightVelocity"=0.0, "Angle"=0.0, "Location"={0.0, 0.0}} ("SensorData"), "LeftVelocity"=w291, "RightVelocity"=w290, "Angle"=w289, "Location"=w288) -> (w292:T16)  [unwired: 2 in]
        n146 = call "PurePursuit.vi"("RobotNeededPathData"=w296, "SensorData"=w292, "Trackwidth"=w282, "Reset"=w285, "Gains"="Gains") -> ("LeftValue"=w295:dbl, "RightValue"=w294:dbl, "Done"=w293:bool)  [unwired: 6 in, 2 out]
      }
    }
    n147 = call "Drive Check for New Command.vi"("input cluster"=w150, "Wait time (ms)"=w137, "Finished?"=w126) -> ("Completion"=w131:T8, "Subsystem Name"=w130:string, "Current Command"=w129:T4, "Initial Trace String"=w128:string, "Next Command"=w152:T18)  [unwired: 4 in]
    n148 = local write "Right Output"(w132) -> ()
    n149 = local write "Left Output"(w127) -> ()
    n150 = case shown="True" w126 {
      frame False {
      }
      frame True {
        n151 = global write "Drive Published Globals.vi" "Drive Done"(TRUE ("Command Done")) -> ()
      }
    }
    n152 = case shown="\"Successful\", \"Aborted\"" w131 {
      selector: w131 -> [_ w162]
      tunnel: w128 -> [_ w157]
      tunnel: w129 -> [_ w158]
      tunnel: w130 -> [_ w154]
      frame "Incomplete", Default {
        # "Continuing current command"
      }
      frame "Successful", "Aborted" {
        # "Report and setup for next command"
        n153 = Unbundle By Name(w158) -> ("Left Speed"=w160:dbl, "Right Speed"=w161:dbl, "Duration"=w155:dbl)
        n154 = Format Into String(format string="L %.1f, R %.1f, D %f", initial string=w157, w160, w161, w155) -> (resulting string=w156:string)  [unwired: 1 in, 1 out]
        "Current\nCmd" <- w156
        n155 = call <vilib>:"Trace Results.vi"("Status of previous command"=w162, "Description"=w156, "Subsystem"=w154) -> ()  [unwired: 9 in]
      }
    }
  }
